vi "Qualified Name - When Constructed - Returns Configured Value.vi"() -> ()   [LabVIEW 2017, in "Test Case.Tests.lvlib"]
uses:
  Test Case.Tests.lvlib
  Test Case/Test Case.lvclass/Test Case.ctl
  Test Case/Get Qualified Name.vi
  Test Case/Test Case.lvclass
  <vilib>/PNR/Transparent Assertions/Transparent Assertions/Transparent Assertions.lvlib
panel:
  out "error out":errorcluster
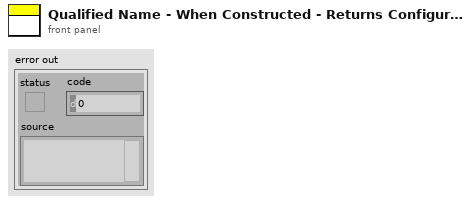
[diagram p1: front panel]
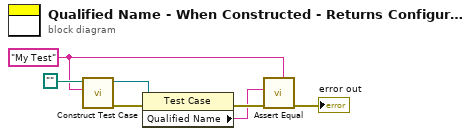
[diagram p0: block diagram]
diagram:
  w1 = "My Test" ("Qualified Name")
  n1 = call "Construct Test Case.vi"("Qualified Name"=w1, "Path"=path "") -> ("error out"=w7:errorcluster, "Test Case out"=w4:refnum<class "Test Case.lvclass">)  [unwired: 8 in]
  n2 = property class="Test Case"(reference=w4, error in=w7) -> (error out=w5:errorcluster, "Qualified Name"=w3:string)  [unwired: 1 out]
  n3 = call <vilib>:"Assert Equal.vi"("Expected"=w1, "error in (no error)"=w5, "Actual"=w3) -> ("error out"=→"error out":errorcluster)  [unwired: 8 in]
